vi "SP SP - set value DBL.vi"(8 "error in (no error)":errorcluster, 11 "JSON string":string) -> (0 "error out":errorcluster, 3 "value":string)   [LabVIEW 2020, in "ui-testing.lvlib"]
doc: "copyright: Thomas Zilliox©"
uses:
  ui-testing.lvlib
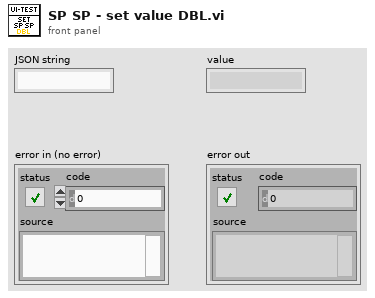
[diagram p1: front panel]
types:
  T1 = cluster{"control":string, "subpanel":string, "subsubpanel":string, "value":dbl}
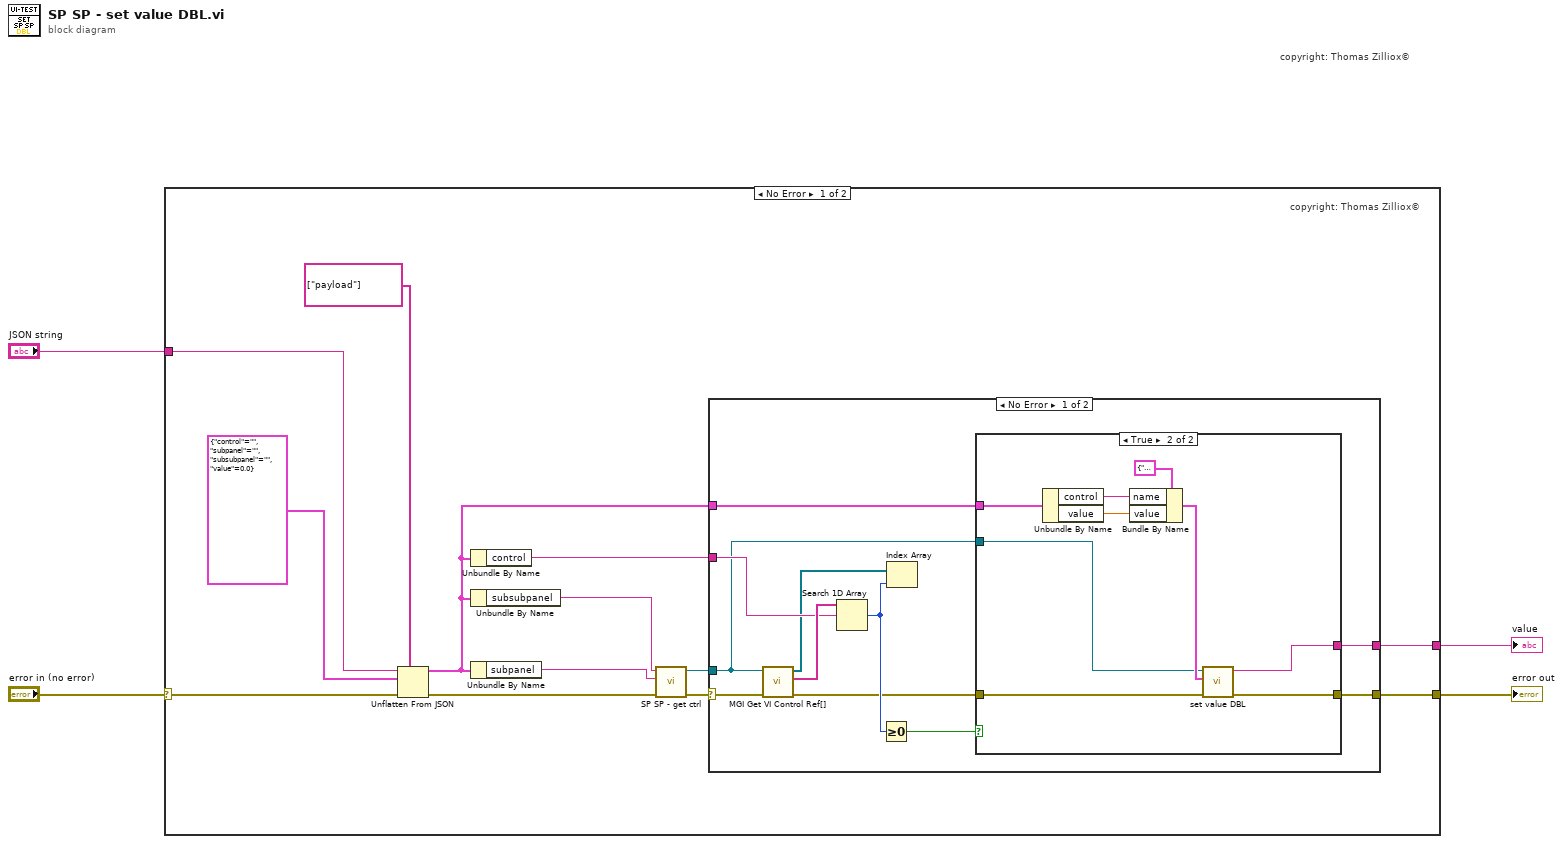
[diagram p0: block diagram]
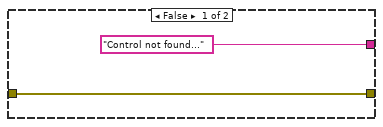
[diagram p2: hidden frame]
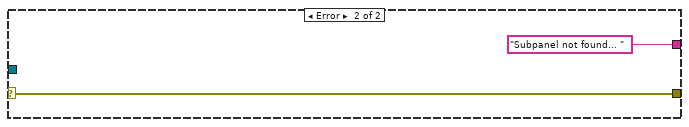
[diagram p3: hidden frame]
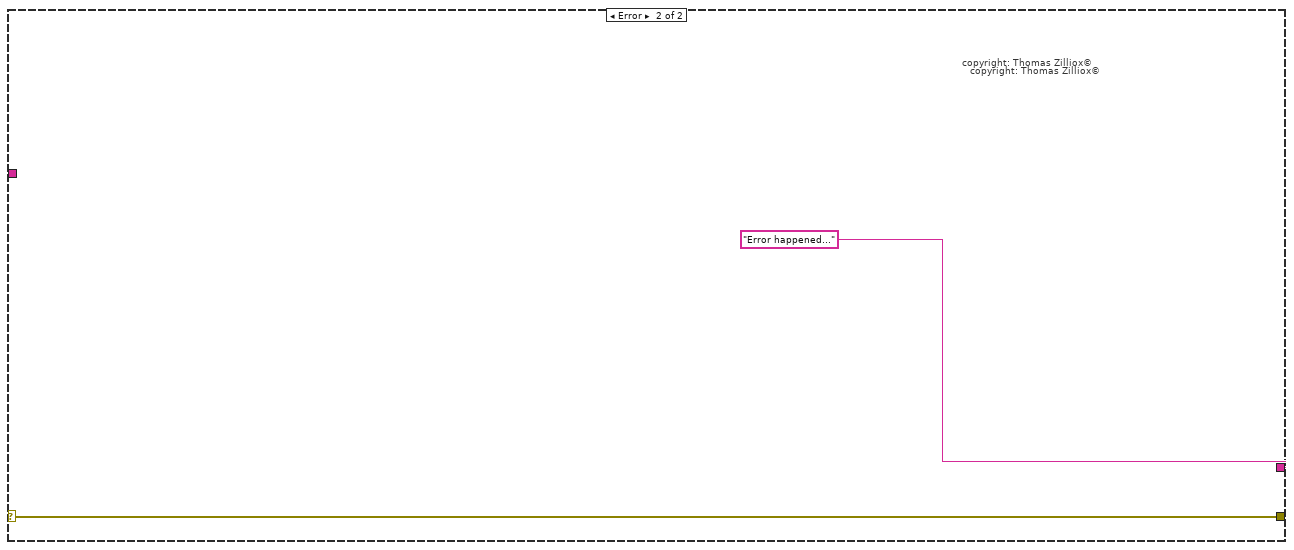
[diagram p4: hidden frame]
diagram:
  # "copyright: Thomas Zilliox©"
  n1 = case shown="No Error" "error in (no error)" {
    selector: "error in (no error)" -> [w13 w43]
    tunnel: "JSON string" -> [w15 _]
    tunnel: [w14 w43] -> w3
    tunnel: [w12 "Error happened..."] -> w1
    frame No Error {
      # "copyright: Thomas Zilliox©"
      n2 = Unflatten From JSON(path=string[] ["payload"], JSON string=w15, type and defaults=T1 {"control"="", "subpanel"="", "subsubpanel"="", "value"=0.0}, error in (no error)=w13) -> (value=w9:T1, error out=w16:errorcluster)  [unwired: 3 in]
      n3 = Unbundle By Name(w9) -> ("control"=w10:string)
      n4 = Unbundle By Name(w9) -> ("subsubpanel"=w8:string)
      n5 = Unbundle By Name(w9) -> ("subpanel"=w7:string)
      n6 = call "SP SP - get ctrl.vi"("error in (no error)"=w16, "subpanel"=w7, "subsubpanel"=w8) -> ("error out"=w5:errorcluster, "VI out"=w6:refnum<vi>)  [unwired: 6 in, 1 out]
      n7 = case shown="No Error" w5 {
        selector: w5 -> [w18 w40]
        tunnel: [w28 w40] -> w14
        tunnel: w6 -> [w19 _]
        tunnel: w10 -> [w25 _]
        tunnel: [w27 "Subpanel not found... " ("result string")] -> w12
        tunnel: w9 -> [w20 _]
        frame No Error {
          n8 = call <userlib>:"MGI Get VI Control Ref[].vi"("error in"=w18, "VI (Caller)"=w19) -> ("error out"=w22:errorcluster, "Control Label Chain[i]"=w26:string[], "Control[i]"=w24:refnum<vi>[])  [unwired: 6 in, 1 out]
          n9 = Search 1D Array(1D array=w26, element=w25) -> (index of element=w23:i32)  [unwired: 1 in]
          n10 = Greater Or Equal To 0?(x=w23) -> (x >= 0?=w21:bool)
          n11 = Index Array(array=w24, index=w23) -> ()  [unwired: 1 out]
          n12 = case shown="True" w21 {
            tunnel: w22 -> [w30 w33]
            tunnel: [w30 w31] -> w28
            tunnel: ["Control not found..." ("result string") w32] -> w27
            tunnel: w20 -> [_ w35]
            tunnel: w19 -> [_ w34]
            frame False {
            }
            frame True {
              n13 = Unbundle By Name(w35) -> ("control"=w36:string, "value"=w37:dbl)
              n14 = Bundle By Name(cluster=cluster{"name":string, "value":dbl} {"name"="", "value"=0.0} ("Payload"), "name"=w36, "value"=w37) -> (w38:cluster{"name":string, "value":dbl})
              n15 = call "set value DBL.vi"("error in (no error)"=w33, "Payload"=w38, "VI Ref"=w34) -> ("error out"=w31:errorcluster, "return value"=w32:string)  [unwired: 7 in]
            }
          }
        }
        frame Error {
        }
      }
    }
    frame Error {
      # "copyright: Thomas Zilliox©"
      # "copyright: Thomas Zilliox©"
    }
  }
  "error out" <- w3
  "value" <- w1
